vi "Settings Dialog.vi"(8 "error in (no error)":errorcluster, 11 "Settings in":T1={"Hardware Configuration"={"DAQmx Channel"="", "Max Input"=10.0, "Min Input"=-10.0, "Sample Rate"=1000.0, "DAQmx Task"=""}, "Logging Configuration"={"Log File Base Path"=path "", "TDMS File Reference"=refnum, "Samples to Save"=0, "Trigger - Time"=0, "Trigger - Threshold"=0.0, "Trigger - Channel"=0, "Enable Time Trigger"=FALSE, "Enable Threshold Trigger"=FALSE, "Always Log"=FALSE}}) -> (0 "error out":errorcluster, 1 "Cancelled?":bool=TRUE, 2 "UI Refresh Needed?":bool, 3 "Settings out":T1={"Hardware Configuration"={"DAQmx Channel"="", "Max Input"=10.0, "Min Input"=-10.0, "Sample Rate"=1000.0, "DAQmx Task"=""}, "Logging Configuration"={"Log File Base Path"=path "C:/Users/jpassiak/Documents/LabVIEW Data/Logged Data.tdms", "TDMS File Reference"=refnum, "Samples to Save"=0, "Trigger - Time"=0, "Trigger - Threshold"=0.0, "Trigger - Channel"=0, "Enable Time Trigger"=FALSE, "Enable Threshold Trigger"=FALSE, "Always Log"=FALSE}})   [LabVIEW 2016, in "Settings.lvlib"]
doc: "Dialog for selecting user specified settings."
uses:
  Settings.lvlib
  Settings.ctl
  Acquisition/Hardware Configuration.ctl
  Logging/Logging Configuration.ctl
  <vilib>/Utility/xml.llb/Write to XML File(string).vi
  Acquisition/Acquisition.lvlib
  Logging/Logging.lvlib
panel:
  in  "Channel - description":string
  in  "User":string
  in  "Data - description":string
  in  "Sample Rate (Hz)":dbl=1000.0
  in  "Min Input (V)":dbl=-10.0
  in  "Max Input (V)":dbl=10.0
  in  "Acquisition channels":tag="Dev1/ai0"
  in  "Log File Path":path
  in  "Cancel Button":bool
  in  "OK Button":bool
  # "Non visible portion of dialog (needed for connector pane)."
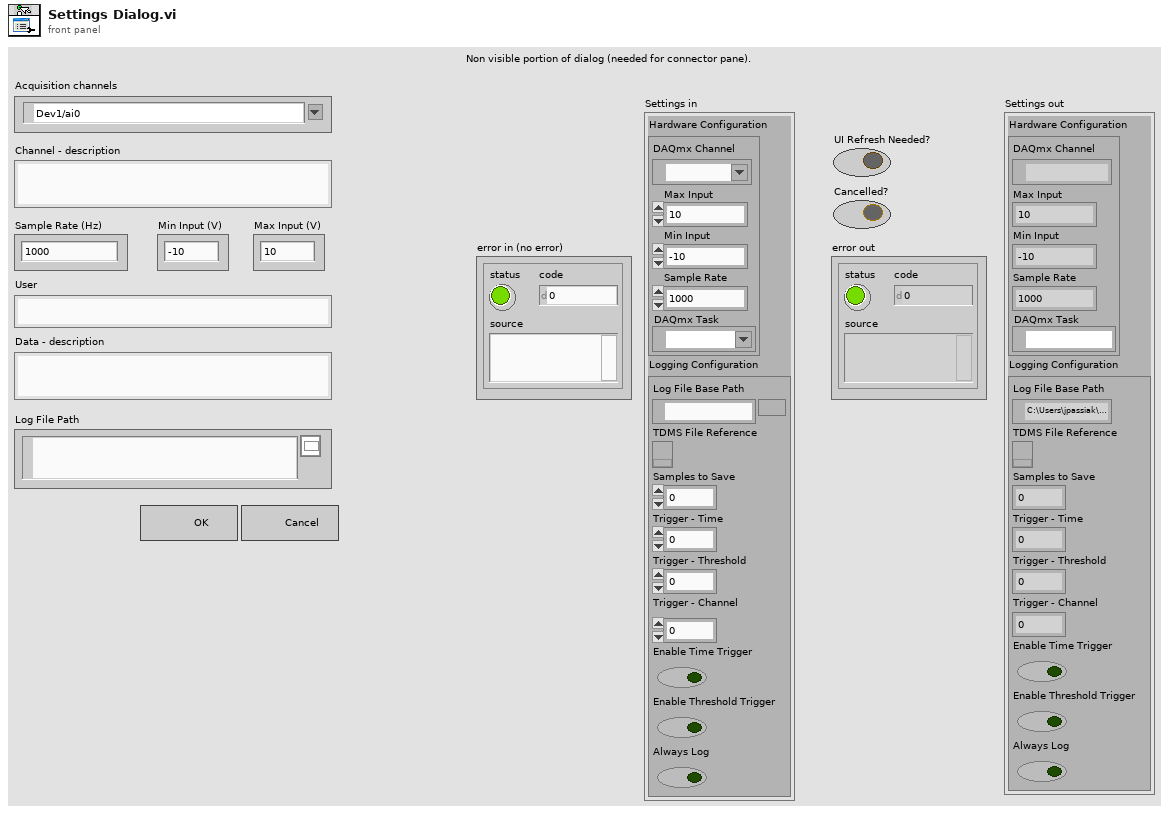
[diagram p1: front panel]
types:
  T1 = typedef "Settings.lvlib/Settings.ctl" = cluster{"Hardware Configuration":T2, "Logging Configuration":T3}
  T2 = typedef "Acquisition.lvlib/Hardware Configuration.ctl" = cluster{"DAQmx Channel":tag, "Max Input":dbl, "Min Input":dbl, "Sample Rate":dbl, "DAQmx Task":refnum<k21>}
  T3 = typedef "Logging.lvlib/Logging Configuration.ctl" = cluster{"Log File Base Path":path, "TDMS File Reference":refnum<k34>, "Samples to Save":u32, "Trigger - Time":u32, "Trigger - Threshold":dbl, "Trigger - Channel":u32, "Enable Time Trigger":bool, "Enable Threshold Trigger":bool, "Always Log":bool}
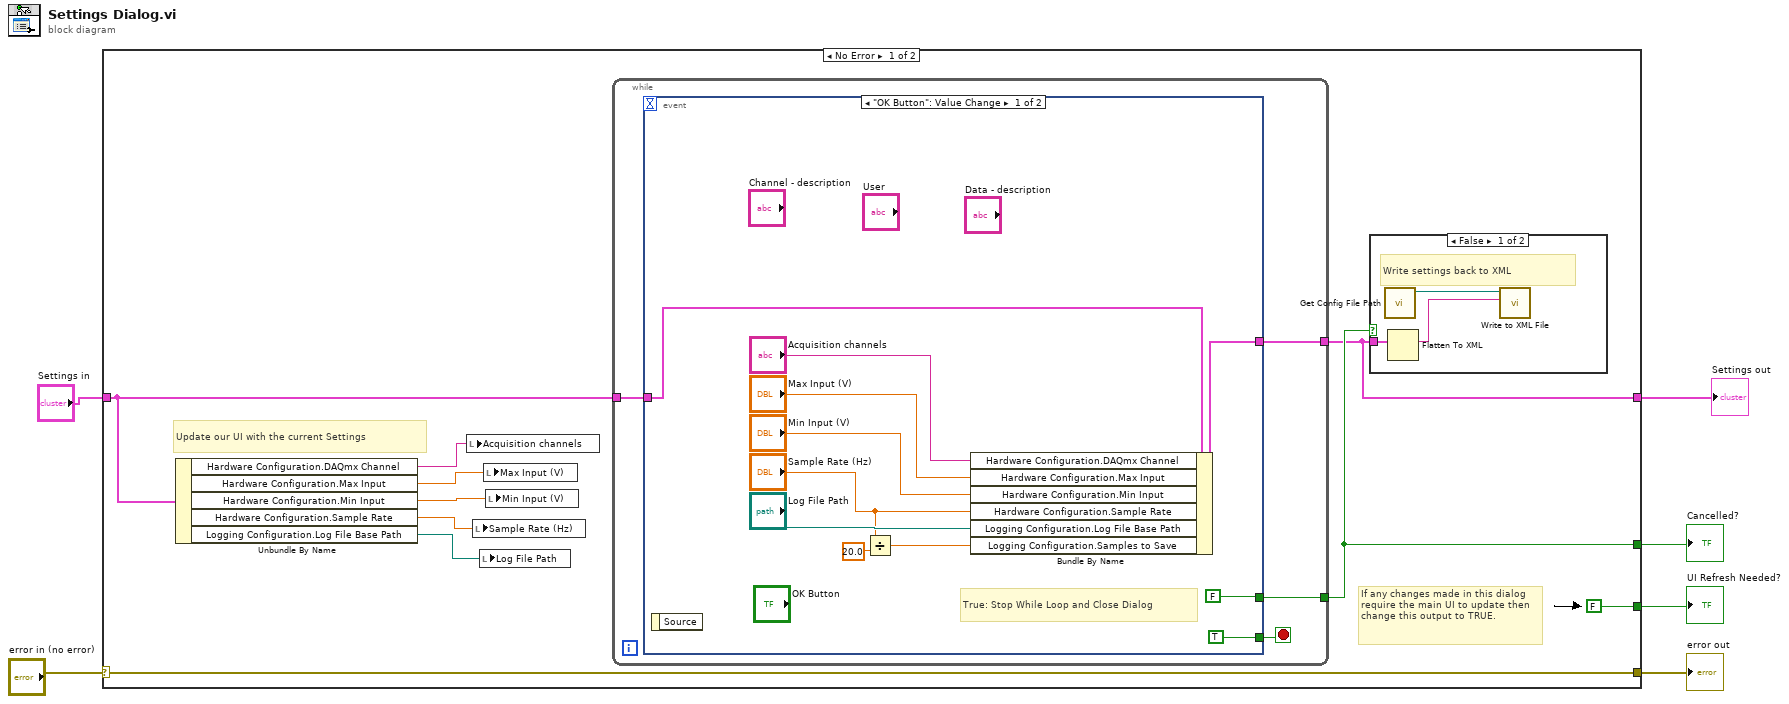
[diagram p0: block diagram]
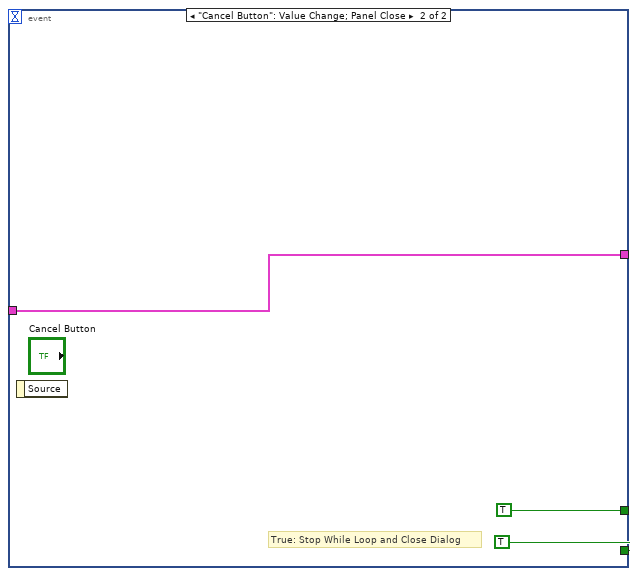
[diagram p2: hidden frame]
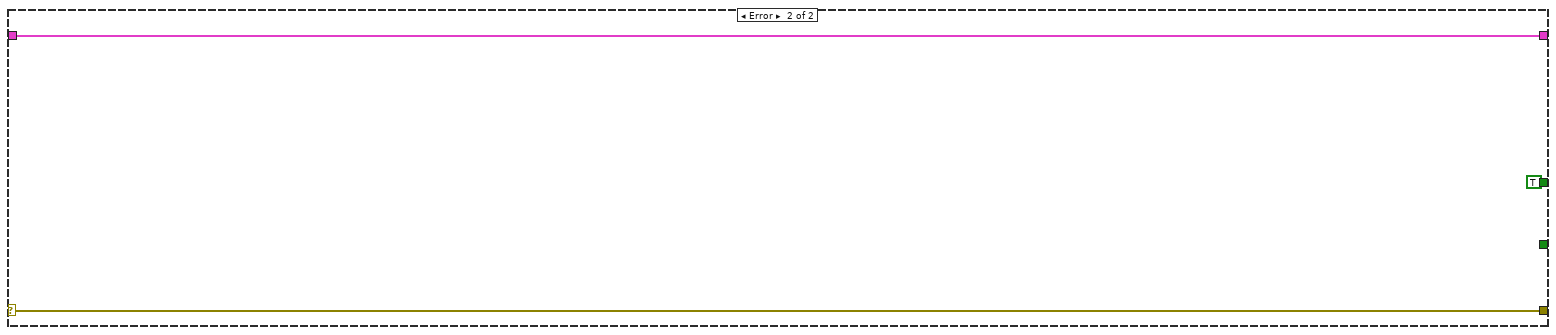
[diagram p4: hidden frame]
diagram:
  n1 = case shown="No Error" "error in (no error)" {
    selector: "error in (no error)" -> [w16 w40]
    tunnel: [w16 w40] -> w6
    tunnel: "Settings in" -> [w7 w39]
    tunnel: [w13 w39] -> w1
    tunnel: [FALSE ("UI Refresh Needed?") _] -> w5
    tunnel: [w14 TRUE ("UI Refresh Needed?")] -> w4
    frame No Error {
      # "Update our UI with the current Settings"
      # "If any changes made in this dialog require the main UI to update then change this output to TRUE."
      n2 = Unbundle By Name(w7) -> ("Hardware Configuration.DAQmx Channel"=w9:tag, "Hardware Configuration.Max Input"=w10:dbl, "Hardware Configuration.Min Input"=w11:dbl, "Hardware Configuration.Sample Rate"=w12:dbl, "Logging Configuration.Log File Base Path"=w8:path)
      n3 = local write "Acquisition channels"(w9) -> ()
      n4 = local write "Sample Rate (Hz)"(w12) -> ()
      n5 = local write "Log File Path"(w8) -> ()
      n6 = local write "Max Input (V)"(w10) -> ()
      n7 = local write "Min Input (V)"(w11) -> ()
      n8 = while {
        tunnel: [w20] -> w14
        tunnel: [w19] -> w13
        tunnel: w7 -> [w18]
        stop <- w17 stop-if-true
        n9 = event shown="[0] \"OK Button\": Value Change" {
          selector: _ -> [_ _]
          dyn-events: _ -> [_ _]
          timeout: _ -> [_ _]
          tunnel: [w29 w34] -> w19
          tunnel: w18 -> [w28 w34]
          tunnel: [FALSE ("UI Refresh Needed?") TRUE ("UI Refresh Needed?")] -> w20
          tunnel: [TRUE TRUE] -> w17
          event "OK Button": Value Change {
            # "True: Stop While Loop and Close Dialog"
            n10 = event-data() -> ()  [unwired: 1 in, 1 out]
            n11 = Divide(x="Sample Rate (Hz)", y=20.0) -> (x/y=w22:dbl)
            n12 = Bundle By Name(cluster=w28, "Hardware Configuration.DAQmx Channel"="Acquisition channels", "Hardware Configuration.Max Input"="Max Input (V)", "Hardware Configuration.Min Input"="Min Input (V)", "Hardware Configuration.Sample Rate"="Sample Rate (Hz)", "Logging Configuration.Log File Base Path"="Log File Path", "Logging Configuration.Samples to Save"=w22) -> (w29:T1)
          }
          event "Cancel Button": Value Change; Panel Close {
            # "True: Stop While Loop and Close Dialog"
            n13 = event-data() -> ()  [unwired: 1 in, 1 out]
          }
        }
      }
      n14 = case shown="False" w14 {
        tunnel: w13 -> [w36 _]
        frame False {
          # "Write settings back to XML"
          n15 = call "Get Config File Path.vi"() -> ("XML File Path"=w37:path)  [unwired: 10 in, 1 out]
          n16 = Flatten To XML(anything=w36) -> (xml string=w35:string)
          n17 = call-poly <vilib>:"Write to XML File.vi"("XML Input"=w35, "XML File Path"=w37) -> ()  [unwired: 7 in, 3 out]
        }
        frame True {
        }
      }
    }
    frame Error {
    }
  }
  "UI Refresh Needed?" <- w5
  "error out" <- w6
  "Settings out" <- w1
  "Cancelled?" <- w4
